vi "Update Control Refnum Map.vi"(8 "error in (no error)":errorcluster, 11 "Client - Data In":T1) -> (0 "error out":errorcluster, 3 "Client - Data Out":T1)   [LabVIEW 2024]
doc: "Updates the URL and the front panel control refnum map for the client."
uses:
  Controls/Client/Client - Data.ctl
  Shared/Message Queue/Client Message Queues.ctl
  Shared/Message Queue/Message Cluster.ctl
  Shared/Message Queue.lvlib
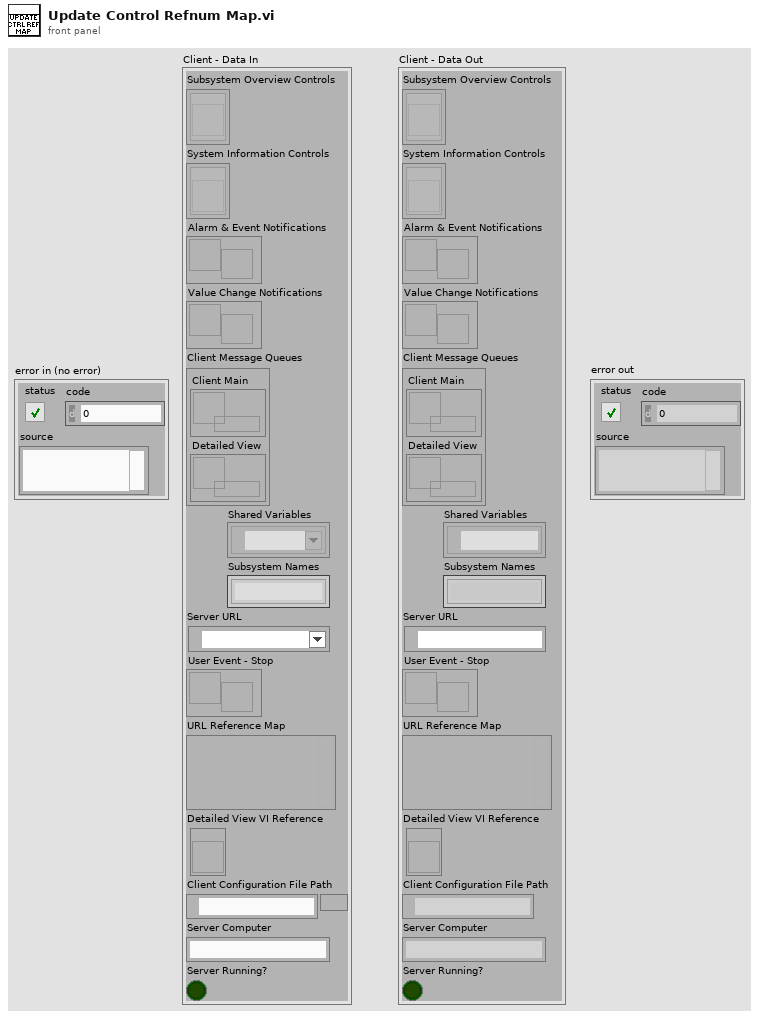
[diagram p1: front panel]
types:
  T1 = typedef "Client - Data.ctl" = cluster{"Subsystem Overview Controls":refnum<vi>[], "System Information Controls":refnum<vi>[], "Alarm & Event Notifications":refnum<user-event>, "Value Change Notifications":refnum<user-event>, "Client Message Queues":T2, "Shared Variables":refnum<k21>[], "Subsystem Names":string[], "Server URL":refnum<k21>, "User Event - Stop":refnum<user-event>, "URL Reference Map":variant, "Detailed View VI Reference":refnum<vi>, "Client Configuration File Path":path, "Server Computer":string, "Server Running?":bool}
  T2 = typedef "Message Queue.lvlib/Client Message Queues.ctl" = cluster{"Client Main":refnum<queue>, "Detailed View":refnum<queue>}
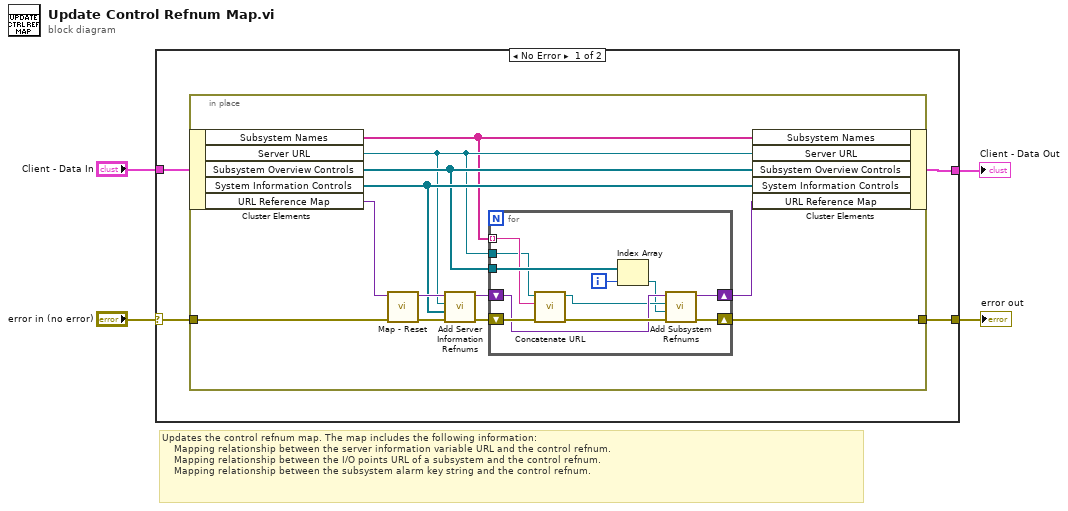
[diagram p0: block diagram]
diagram:
  # "Updates the control refnum map. The map includes the following information:\n    Mapping relationship between the server information variable URL and the control refnum.\n    Mapping relationship between the I/O points URL of a subsystem and the control refnum.\n    Mapping relationship between the subsystem alarm key string and the control refnum."
  n1 = case shown="No Error" "error in (no error)" {
    selector: "error in (no error)" -> [w8 w33]
    tunnel: [w5 w33] -> w3
    tunnel: "Client - Data In" -> [w7 w32]
    tunnel: [w6 w32] -> w1
    frame No Error {
      n2 = in-place {
        in-place-border: [w10] -> w5
        in-place-border: w8 -> [w9]
        n3 = in-place-cluster #1(w7) -> ("Subsystem Names"=w11:string[], "Server URL"=w12:refnum<k21>, "Subsystem Overview Controls"=w13:refnum<vi>[], "System Information Controls"=w14:refnum<vi>[], "URL Reference Map"=w15:variant)
        n4 = call "Map - Reset.vi"("error in (no error)"=w9, "Map In"=w15) -> ("error out"=w16:errorcluster, "Map Out"=w17:variant)  [unwired: 8 in]
        n5 = call "Add Server Information Refnums.vi"("error in (no error)"=w16, "Server Information Controls"=w14, "Server URL"=w12, "Map In"=w17) -> ("error out"=w19:errorcluster, "Map Out"=w20:variant)  [unwired: 6 in]
        n6 = for {
          shift-right: [w29] -> w10
          shift-left: w19 -> [w30]
          shift-right: [w27] -> w18
          shift-left: w20 -> [w28]
          tunnel: w13 -> [w26]
          tunnel: w12 -> [w22]
          tunnel: w11 -> [w23] mode=indexing
          i -> [w25]
          n7 = call "Concatenate URL.vi"("error in (no error)"=w30, "Child Name"=w23, "Parent URL"=w22) -> ("error out"=w31:errorcluster, "Child URL"=w24:refnum<k21>)  [unwired: 7 in]
          n8 = Index Array(array=w26, index=w25) -> (element=w21:refnum<vi>)
          n9 = call "Add Subsystem Refnums.vi"("error in (no error)"=w31, "Subsystem Overview Control"=w21, "Subsystem URL"=w24, "Map In"=w28) -> ("error out"=w29:errorcluster, "Map Out"=w27:variant)  [unwired: 6 in]
        }
        n10 = in-place-cluster #1("Subsystem Names"=w11, "Server URL"=w12, "Subsystem Overview Controls"=w13, "System Information Controls"=w14, "URL Reference Map"=w18) -> (w6:T1)
      }
    }
    frame Error {
    }
  }
  "error out" <- w3
  "Client - Data Out" <- w1
